vi "Generate Variable Name.vi"(10 "Default Name":string="Var", 11 "Variables":cluster{"Name":string, "Value":variant}[](array[cluster])) -> (3 "Name":string)   [LabVIEW 2015, in "Project.lvclass"]
uses:
  Project.lvclass
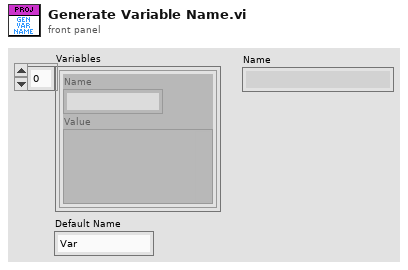
[diagram p1: front panel]
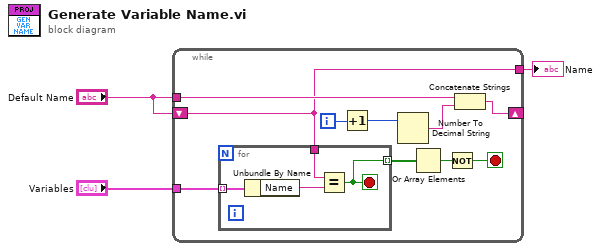
[diagram p0: block diagram]
diagram:
  n1 = while {
    tunnel: "Variables" -> [w13]
    shift-right: [w9] -> _
    shift-left: "Default Name" -> [w5]
    tunnel: "Default Name" -> [w6]
    tunnel: [w5] -> w2
    i -> [w11]
    stop <- w7 stop-if-true
    n2 = for {
      tunnel: w13 -> [w15] mode=indexing
      tunnel: w5 -> [w17]
      tunnel: [w16] -> w12 mode=indexing
      stop <- w16 stop-if-true
      n3 = Unbundle By Name(w15) -> ("Name"=w14:string)
      n4 = Equal?(x=w17, y=w14) -> (x = y?=w16:bool)
    }
    n5 = Increment(x=w11) -> (x+1=w10:i32)
    n6 = Number To Decimal String(number=w10) -> (decimal integer string=w4:string)  [unwired: 1 in]
    n7 = Or Array Elements(Boolean array=w12) -> (logical OR=w8:bool)
    n8 = Not(x=w8) -> (.not. x?=w7:bool)
    n9 = Concatenate Strings(w6, w4) -> (w9:string)
  }
  "Name" <- w2
